vi "Read_Tirf.vi"(3 "Display":bool=TRUE, 4 "Averages":i32=1 min=1, 5 "Tirf-Handle":i32) -> (0 "coerced(sum)":dbl, 1 "coerced(y)":dbl, 2 "coerced(x)":dbl)   [LabVIEW 2019]
uses:
  Dependencies/TIRF-Lock.dll
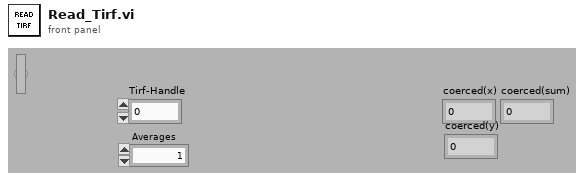
[diagram p1: front panel]
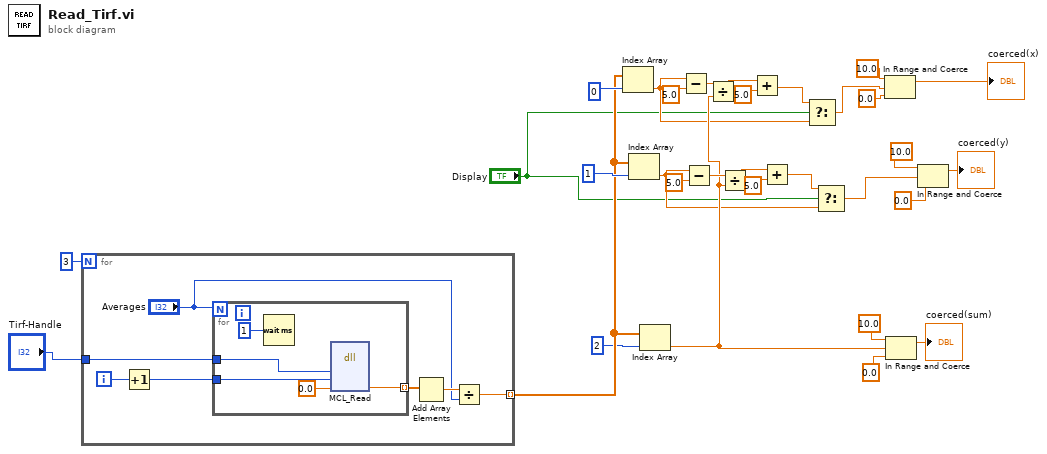
[diagram p0: block diagram]
diagram:
  n1 = for {
    N: 3 -> [_]
    tunnel: [w35] -> w13 mode=indexing
    tunnel: "Tirf-Handle" -> [w32]
    i -> [w33]
    n2 = Increment(x=w33) -> (x+1=w34:i32)
    n3 = for {
      N: "Averages" -> [_]
      tunnel: w32 -> [w40]
      tunnel: [w42] -> w37 mode=indexing
      tunnel: w34 -> [w41]
      n4 = Wait (ms)(milliseconds to wait=1) -> ()  [unwired: 1 out]
      n5 = dll-call lib="E:/DevHardSoftware/MMicroscopy/HardwareAdapter/Stages/Dependencies/TIRF-Lock.dll" fn="MCL_Read" label="tirf read"("handle"=w40, "axis"=w41, "readValue"=0.0) -> ("readValue"=w42:dbl)  [unwired: 5 in, 3 out]
    }
    n6 = Add Array Elements(numeric array=w37) -> (sum=w38:dbl)
    n7 = Divide(x=w38, y="Averages") -> (x/y=w35:dbl)
  }
  n8 = Index Array(array=w13, index=0) -> (element=w5:dbl)
  n9 = Index Array(array=w13, index=1) -> (element=w2:dbl)
  n10 = Index Array(array=w13, index=2) -> (element=w11:dbl)
  n11 = Subtract(x=w5, y=5.0) -> (x-y=w30:dbl)
  n12 = Subtract(x=w2, y=5.0) -> (x-y=w22:dbl)
  n13 = Divide(x=w30, y=w11) -> (x/y=w27:dbl)
  n14 = Divide(x=w22, y=w11) -> (x/y=w20:dbl)
  n15 = Add(x=w27, y=5.0) -> (x+y=w7:dbl)
  n16 = Add(x=w20, y=5.0) -> (x+y=w4:dbl)
  n17 = Select(t=w7, s="Display", f=w5) -> (s? t:f=w6:dbl)
  n18 = Select(t=w4, s="Display", f=w2) -> (s? t:f=w3:dbl)
  n19 = In Range and Coerce(upper limit=10.0, x=w6, lower limit=0.0) -> (coerced(x)=→"coerced(x)":dbl)  [unwired: 1 out]
  n20 = In Range and Coerce(upper limit=10.0, x=w11, lower limit=0.0) -> (coerced(x)=→"coerced(sum)":dbl)  [unwired: 1 out]
  n21 = In Range and Coerce(upper limit=10.0, x=w3, lower limit=0.0) -> (coerced(x)=→"coerced(y)":dbl)  [unwired: 1 out]
